vi "KE2410_CommandsGlobal.vi"() -> ()   [LabVIEW 2013, in "KE2410.lvclass"]
uses:
  KE2410.lvclass
panel:
  in  "Keithley 2410 GPIB Setup":T1={"Instrument name"="Keithley 2410", "Command \"Reset\""="*rst", "Command \"Initialise\""=":Calculate:state 0; :trigger:source imm; :trigger:count 1; :route:terminals %s; :format:data ASCii; :format:elements CURR; :trace:tstamp:format delta; :source:voltage:range MAX; :sense:func 'curr:dc'; :sense:current:range:auto 1; :sense:current:prot %1.6f;", "Command \"Arm\""=":outp:stat OFF; :sour:func VOLT; :sour:volt:mode FIX; :sour:volt:lev 0; :outp:stat ON; ", "Command \"SetVolts\""=":sour:volt:lev %4.2f; :sense:current:range:auto 1; :sense:current:prot %1.6f;", "Command \"Compliance?\""=":SENS:CURR:PROT:TRIP?;", "Command \"Standby\""=":sour:volt:lev 0.0; :outp:stat OFF;\n", "Command \"Read Current\""="READ?"}
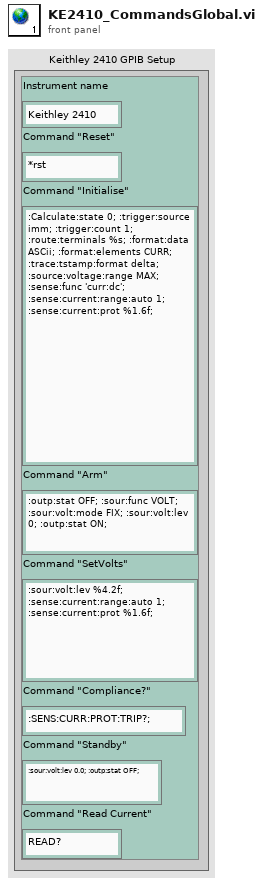
[diagram p1: front panel]
types:
  T1 = cluster{"Instrument name":string, "Command \"Reset\"":string, "Command \"Initialise\"":string, "Command \"Arm\"":string, "Command \"SetVolts\"":string, "Command \"Compliance?\"":string, "Command \"Standby\"":string, "Command \"Read Current\"":string}
diagram:
